vi "main.vi"() -> ()   [LabVIEW 2020]
uses:
  D:/SuperPython-master/ScintillaNET.dll
  ScintillaNET.dll
  <vilib>/picture/picture.llb/imagedata.ctl
  C:/Program Files/National Instruments/LabVIEW 2020/vi.lib/ActorFramework/Actor/Actor.lvclass
  <vilib>/ActorFramework/Message Enqueuer/Message Enqueuer.lvclass/Message Enqueuer.ctl
  <vilib>/ActorFramework/Message Enqueuer/Enqueue.vi
  C:/Program Files/National Instruments/LabVIEW 2020/vi.lib/ActorFramework/Message/Message.lvclass
  <vilib>/ActorFramework/Stop Msg/Stop Msg.lvclass
  <vilib>/ActorFramework/Message Priority Queue/Priority Enqueue.vi
  <vilib>/Utility/cursorutil.llb/Set Cursor (Icon Pict).vi
  <vilib>/Utility/inputDevices.llb/keyboardAcquire.vi
  <vilib>/Utility/inputDevices.llb/closeKeyboard.vi
  D:/SuperPython-master/AutocompleteMenu-ScintillaNET.dll
  AutocompleteMenu-ScintillaNET.dll
  <vilib>/ActorFramework/Actor/Actor.lvclass
panel:
  in  "工具-帮助":bool
  in  "菜单-下载":bool
  in  "切换界面":bool
  in  "工具-执行":bool
  in  "工具-编译":bool
  in  "工具-导出py":bool
  in  "工具-另存为":bool
  in  "工具-保存":bool
  in  "工具-新建":bool
  in  "工具-打开":bool
  in  "交互信息":string[][](array[string])
  in  "关键字":string[][](array[string])
  in  "执行语句":string[][](array[string])
  in  "图片名称":string[][](array[string])
  in  "停止":bool
  in  "界面":enum32{"选项卡 1", "选项卡 2"}(tab)
  out "编译执行状态":refnum<k24>(container) caption="文本程序"
  out "保存状态":string
  out "文本显示":refnum<k24>(container) caption="文本程序"
  in  "图形程序":picture[][](array[picture])
  out "备注":string[][](array[string])
  in  "辅助线":picture
  in  "连接线":picture
  in  "编辑控件类型":bool
  out "编辑控件":bool
  in  "控件类型":cluster{"二维图片":picture, "类型名称":string}[](array[cluster])
  in  "控件列表":T2(array[cluster])
  in  "全部控件":T3(array[cluster])
  in  "状态":refnum<k24>(container)
  in  "文本编辑":refnum<k24>(container)
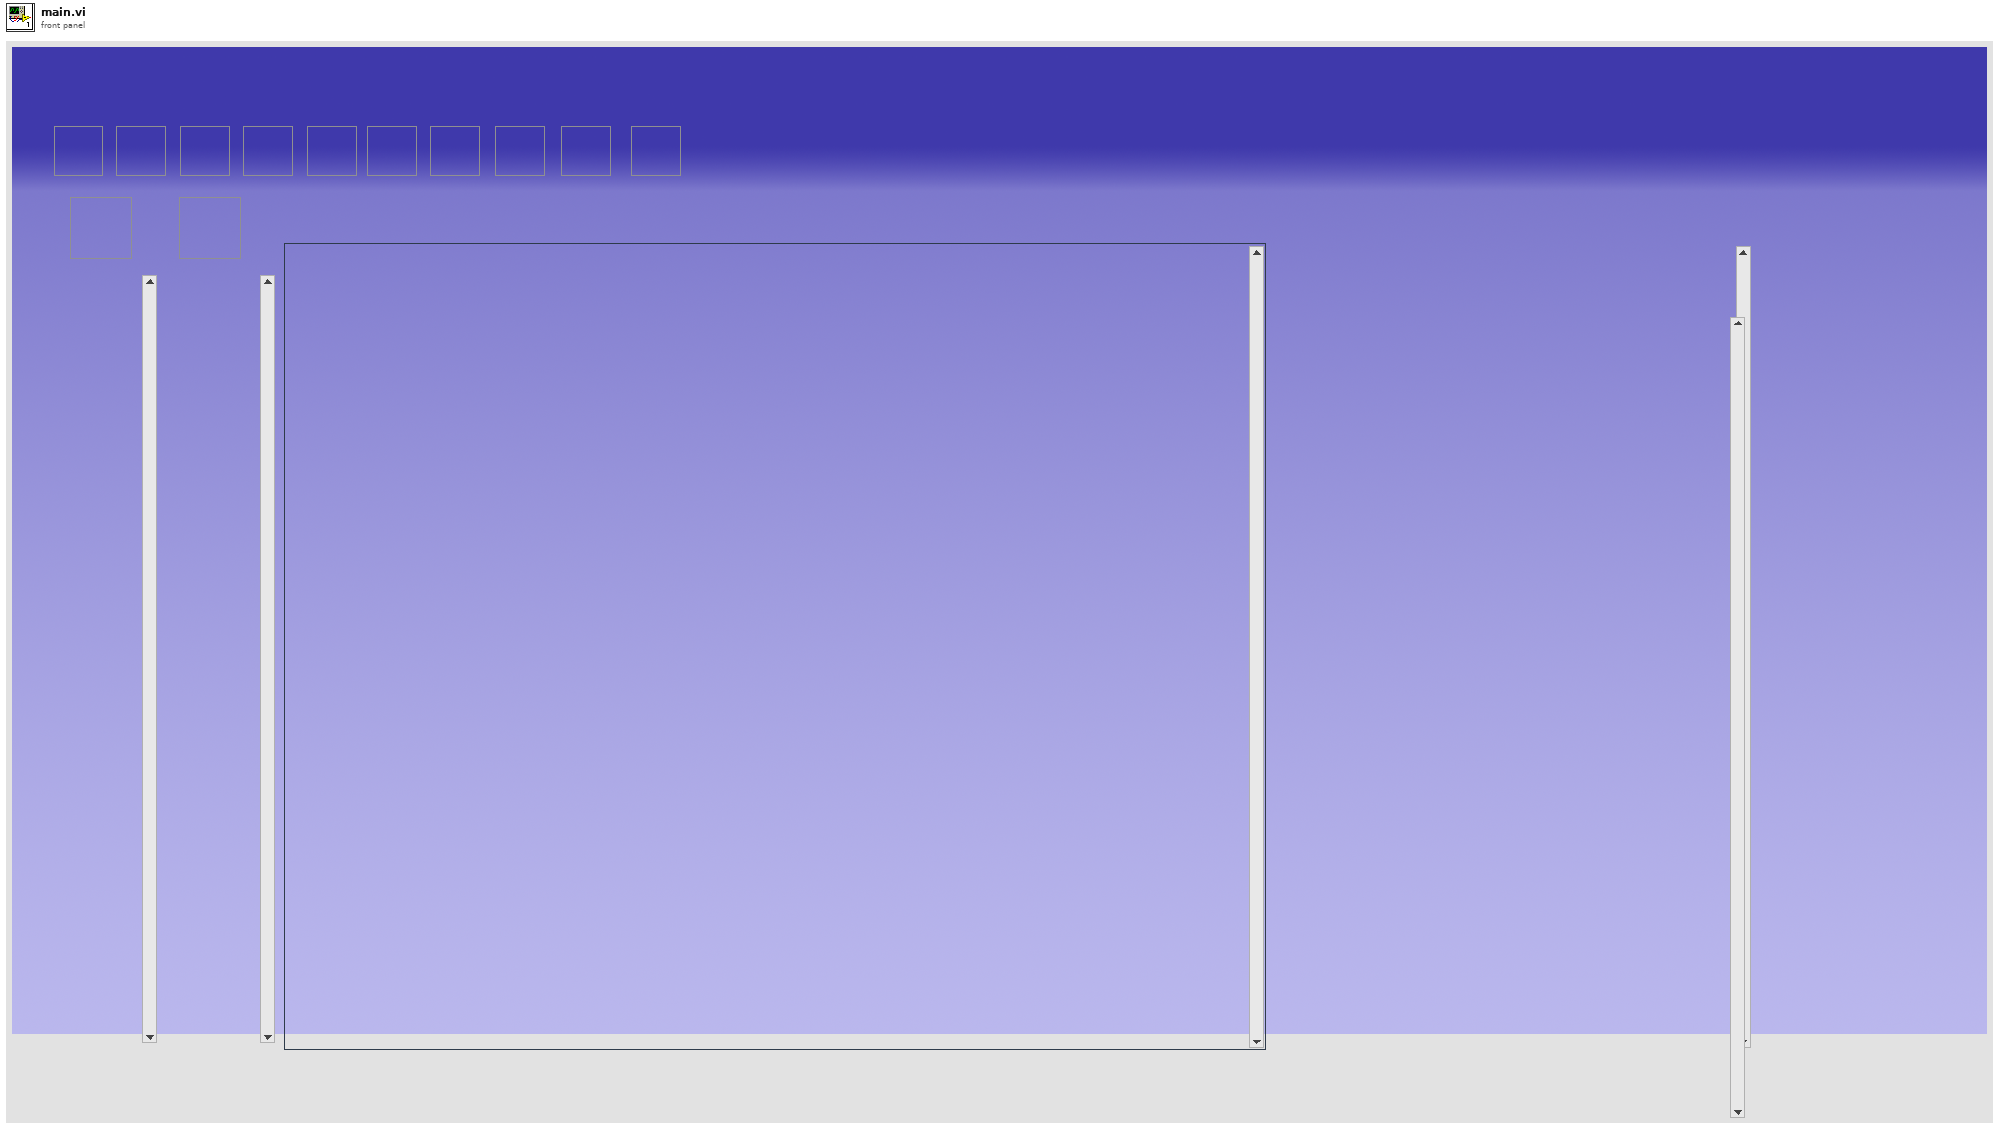
[diagram p1: front panel]
types:
  T1 = typedef "imagedata.ctl" = cluster{"image type":i32, "image depth":i32, "image":u8[], "mask":u8[], "colors":u32[], "Rectangle":cluster{"left":i16, "top":i16, "right":i16, "bottom":i16}}
  T2 = cluster{"图片":picture, "名称":string, "文本程序":string, "关键字":string, "image data":T1}[]
  T3 = cluster{"图片":picture, "名称":string, "文本程序":string, "关键字":string, "image data":T1}[][]
  T4 = cluster{"图形程序":refnum<vi>, "辅助线":refnum<vi>, "图片名称":refnum<vi>, "执行语句":refnum<vi>, "文本程序":refnum<vi>, "控件类型":refnum<vi>, "控件列表":refnum<vi>, "全部控件":refnum<vi>, "关键字":refnum<vi>, "连接线":refnum<vi>, "交互信息":refnum<vi>, "备注":refnum<vi>, "保存状态":refnum<vi>, "VI引用句柄":refnum<vi>, "编译执行状态":refnum<vi>, "TabCtl引用句柄":refnum<vi>, "AXContl":refnum<vi>, "AutoCompele":refnum<k24>, "状态":refnum<vi>}
  T5 = enum16{"0", "1", "2", "3", "4", "5", "6", "7", "8", "9", "A", "B", "C", "D", "E", "F", "G", "H", "I", "J", "K", "L", "M", "N", "O", "P", "Q", "R", "S", "T", "U", "V", "W", "X", "Y", "Z", "F1", "F2", "F3", "F4", "F5", "F6", "F7", "F8", "F9", "F10", "F11", "F12", "F13", "F14", "F15", "ADD", "BACK", "BACKSLASH", "CAPITAL", "COMMA", "DECIMAL", "DELETE", "DIVIDE", "DOWN", "END", "EQUALS", "ESCAPE", "GRAVE (`)", "HOME", "INSERT", "LBRACKET", "LCONTROL", "LEFT", "L ALT", "LSHIFT", "LWIN", "MINUS", "MULTIPLY", "NEXT", "NUMLOCK", "NUMPAD_0", "NUMPAD_1", "NUMPAD_2", "NUMPAD_3", "NUMPAD_4", "NUMPAD_5", "NUMPAD_6", "NUMPAD_7", "NUMPAD_8", "NUMPAD_9", "PAUSE", "PERIOD", "PRIOR (PG UP)", "RBRACKET", "RCONTROL", "RETURN", "RIGHT", "R ALT", "RSHIFT", "RWIN", "SCROLL", "SEMICOLON", "SLASH", "SPACE", "SUBTRACT", "TAB", "UP", "ENTER (num pad)", "' (quote)"}
  T6 = typedef "LVRectTypeDef.ctl" = cluster{"Left":i16, "Top":i16, "Right":i16, "Bottom":i16}
  T7 = typedef "LVPoint32TypeDef.ctl" = cluster{"Horizontal":i32, "Vertical":i32}
  T8 = typedef "LVPositionTypeDef.ctl" = cluster{"Left":i32, "Top":i32}
  T9 = typedef "eventvkey.ctl" = enum16{"ASCII", "Enter", "Return", "Shift", "Ctrl", "Alt", "Cmd", "Opt", "Caps", "NumLock", "Clear", "Break", "Up", "Down", "Left", "Right", "Insert", "Delete", "Home", "End", "PageUp", "PageDown", "Escape", "Help", "Pause", "ScrollLock", "F1", "F2", "F3", "F4", "F5", "F6", "F7", "F8", "F9", "F10", "F11", "F12", "F13", "F14", "F15", "F16", "F17", "F18", "F19", "F20", "F21", "F22", "F23", "F24", "Play", "VolumeUp", "VolumeDown", "Mute", "Two Byte Char"}
  T10 = enum16{"0", "1", "2", "3", "4", "5", "6", "7", "8", "9", "A", "B", "C", "D", "E", "F", "G", "H", "I", "J", "K", "L", "M", "N", "O", "P", "Q", "R", "S", "T", "U", "V", "W", "X", "Y", "Z", "F1", "F2", "F3", "F4", "F5", "F6", "F7", "F8", "F9", "F10", "F11", "F12", "F13", "F14", "F15", "ADD", "BACK", "BACKSLASH", "CAPITAL", "COMMA", "DECIMAL", "DELETE", "DIVIDE", "DOWN", "END", "EQUALS", "ESCAPE", "GRAVE (`)", "HOME", "INSERT", "LBRACKET", "LCONTROL", "LEFT", "L ALT", "LSHIFT", "LWIN", "MINUS", "MULTIPLY", "NEXT", "NUMLOCK", "NUMPAD_0", "NUMPAD_1", "NUMPAD_2", "NUMPAD_3", "NUMPAD_4", "NUMPAD_5", "NUMPAD_6", "NUMPAD_7", "NUMPAD_8", "NUMPAD_9", "PAUSE", "PERIOD", "PRIOR (PG UP)", "RBRACKET", "RCONTROL", "RETURN", "RIGHT", "R ALT", "RSHIFT", "RWIN", "SCROLL", "SEMICOLON", "SLASH", "SPACE", "SUBTRACT", "TAB", "UP", "ENTER (num pad)", "' (quote)"}[]
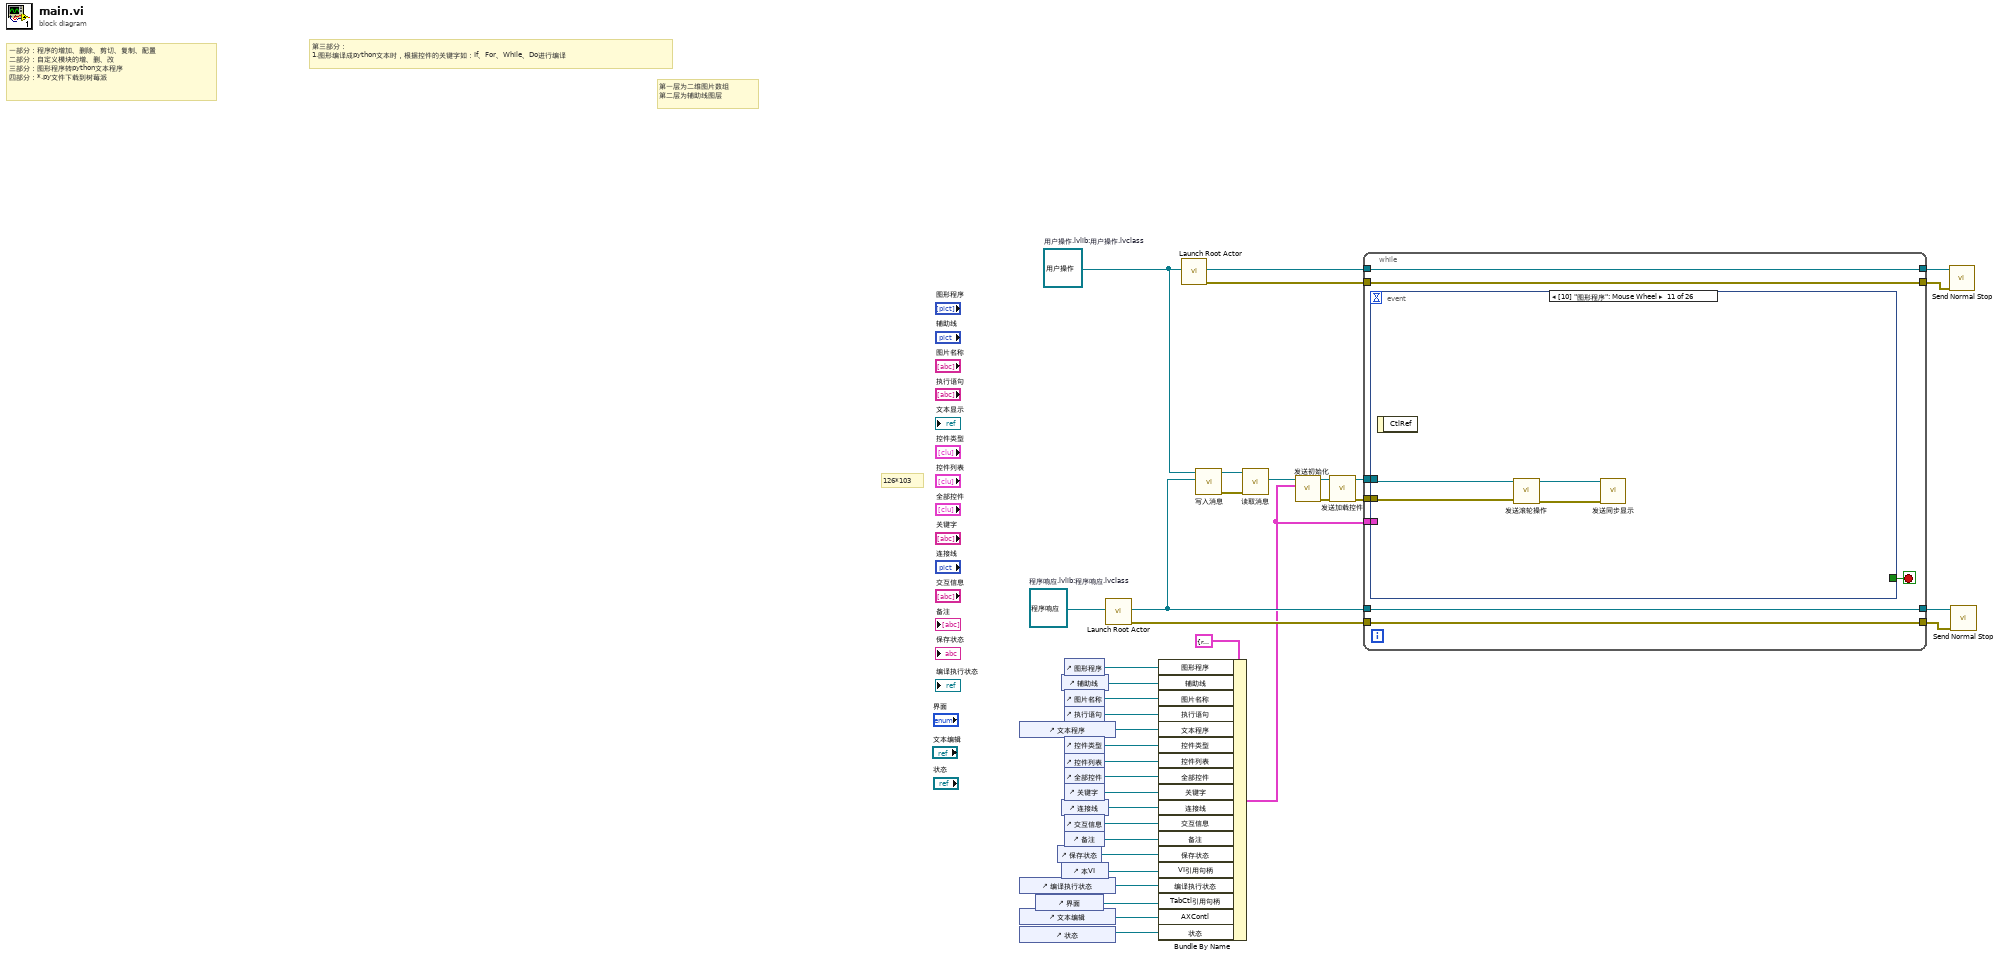
[diagram p0: block diagram]
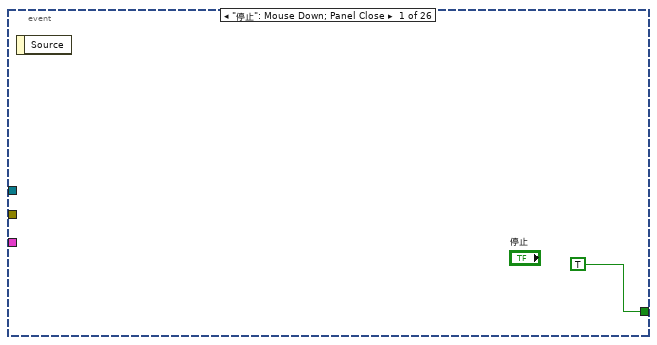
[diagram p2: hidden frame]
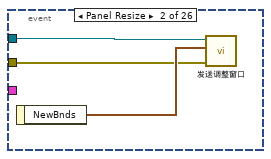
[diagram p3: hidden frame]
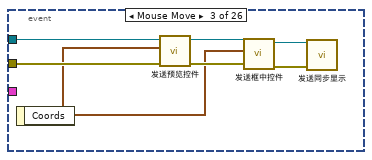
[diagram p4: hidden frame]
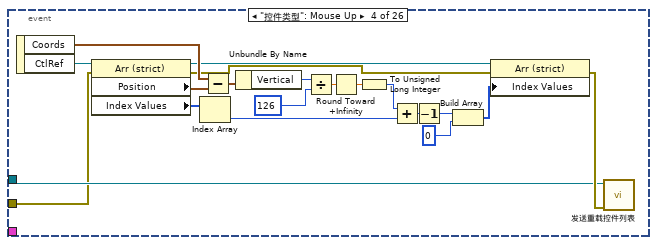
[diagram p5: hidden frame]
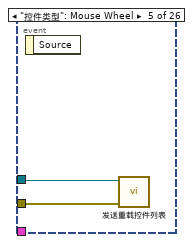
[diagram p6: hidden frame]
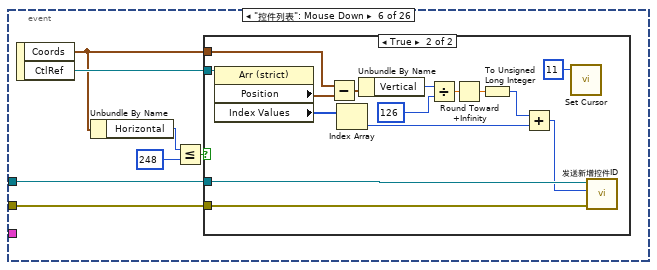
[diagram p7: hidden frame]
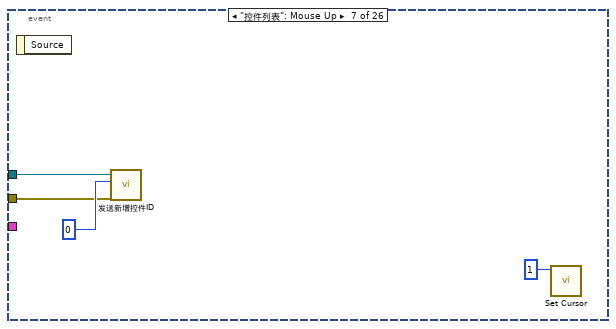
[diagram p9: hidden frame]
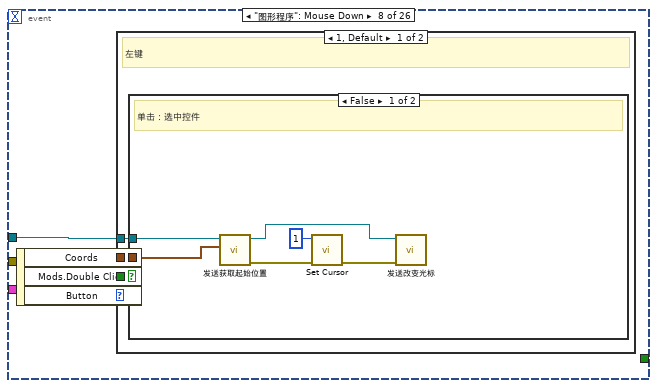
[diagram p10: hidden frame]
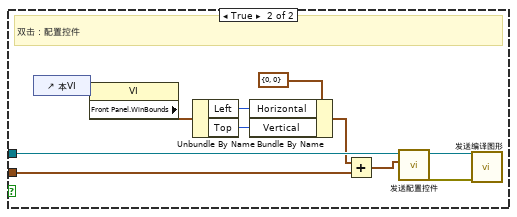
[diagram p11: hidden frame]
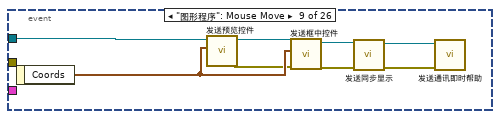
[diagram p13: hidden frame]
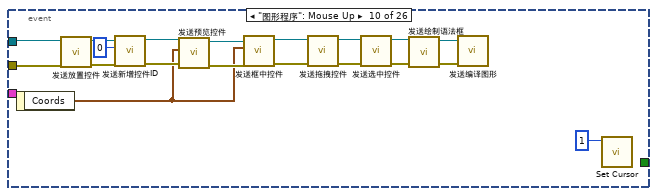
[diagram p14: hidden frame]
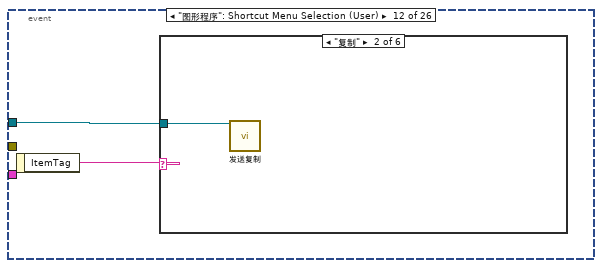
[diagram p15: hidden frame]
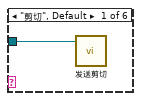
[diagram p16: hidden frame]
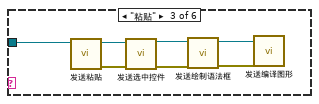
[diagram p17: hidden frame]
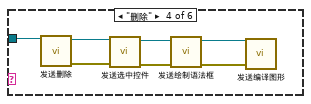
[diagram p18: hidden frame]
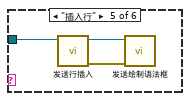
[diagram p19: hidden frame]
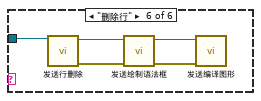
[diagram p20: hidden frame]
diagram:
  w34 = refnum<class "用户操作.lvclass"> refnum  # 用户操作.lvlib:用户操作.lvclass
  w37 = refnum<class "程序响应.lvclass"> refnum  # 程序响应.lvlib:程序响应.lvclass
  # "126*103"
  # "第三部分：\n1.图形编译成python文本时，根据控件的关键字如：If、For、While、Do进行编译"
  # "一部分：程序的增加、删除、剪切、复制、配置\n二部分：自定义模块的增、删、改\n三部分：图形程序转python文本程序\n四部分：*.py文件下载到树莓派"
  # "第一层为二维图片数组\n第二层为辅助线图层"
  n1 = control-ref of="文本程序"() -> (w21:refnum<vi>)
  n2 = control-ref of="编译执行状态"() -> (w13:refnum<vi>)
  n3 = control-ref of="文本编辑"() -> (w10:refnum<vi>)
  n4 = control-ref of="状态"() -> (w5:refnum<vi>)
  n5 = control-ref of="界面"() -> (w11:refnum<vi>)
  n6 = control-ref of="保存状态"() -> (w15:refnum<vi>)
  n7 = control-ref of="辅助线"() -> (w24:refnum<vi>)
  n8 = control-ref of="连接线"() -> (w19:refnum<vi>)
  n9 = control-ref of="本VI"() -> (w14:refnum<vi>)
  n10 = control-ref of="图形程序"() -> (w25:refnum<vi>)
  n11 = control-ref of="图片名称"() -> (w23:refnum<vi>)
  n12 = control-ref of="执行语句"() -> (w22:refnum<vi>)
  n13 = control-ref of="控件类型"() -> (w18:refnum<vi>)
  n14 = control-ref of="控件列表"() -> (w3:refnum<vi>)
  n15 = control-ref of="全部控件"() -> (w2:refnum<vi>)
  n16 = control-ref of="关键字"() -> (w20:refnum<vi>)
  n17 = control-ref of="交互信息"() -> (w17:refnum<vi>)
  n18 = control-ref of="备注"() -> (w16:refnum<vi>)
  n19 = call <vilib>:"Launch Root Actor.vi"("Actor"=w37) -> ("error out"=w29:errorcluster, "Actor's Enqueuer"=w33:refnum<class "Message Enqueuer.lvclass">)  [unwired: 9 in]
  n20 = Bundle By Name(cluster=T4 {"图形程序"=refnum, "辅助线"=refnum, "图片名称"=refnum, "执行语句"=refnum, "文本程序"=refnum, "控件类型"=refnum, "控件列表"=refnum, "全部控件"=refnum, "关键字"=refnum, "连接线"=refnum, "交互信息"=refnum, "备注"=refnum, "保存状态"=refnum, "VI引用句柄"=refnum, "编译执行状态"=refnum, "TabCtl引用句柄"=refnum, "AXContl"=refnum, "AutoCompele"=refnum, "状态"=refnum} ("数据"), "图形程序"=w25, "辅助线"=w24, "图片名称"=w23, "执行语句"=w22, "文本程序"=w21, "控件类型"=w18, "控件列表"=w3, "全部控件"=w2, "关键字"=w20, "连接线"=w19, "交互信息"=w17, "备注"=w16, "保存状态"=w15, "VI引用句柄"=w14, "编译执行状态"=w13, "TabCtl引用句柄"=w11, "AXContl"=w10, "状态"=w5) -> (w1:T4)
  n21 = call <vilib>:"Launch Root Actor.vi"("Actor"=w34) -> ("error out"=w27:errorcluster, "Actor's Enqueuer"=w32:refnum<class "Message Enqueuer.lvclass">)  [unwired: 9 in]
  n22 = call-dynamic "写入消息.vi"("操作者框架:消息待入队列"=w33, "用户操作输入"=w34) -> ("error out"=w35:errorcluster, "用户操作输出"=w36:refnum<class "用户操作.lvclass">)  [unwired: 8 in]
  n23 = call-dynamic "读取消息.vi"("error in (no error)"=w35, "用户操作输入"=w36) -> ("操作者框架:消息待入队列"=w12:refnum<class "Message Enqueuer.lvclass">)  [unwired: 7 in, 2 out]
  n24 = call "发送初始化.vi"("数据"=w1, "Message Enqueuer"=w12) -> ("error out"=w7:errorcluster, "Message Enqueuer out"=w9:refnum<class "Message Enqueuer.lvclass">)  [unwired: 8 in]
  n25 = call "发送加载控件.vi"("error in (no error)"=w7, "Message Enqueuer"=w9) -> ("error out"=w6:errorcluster, "Message Enqueuer out"=w8:refnum<class "Message Enqueuer.lvclass">)  [unwired: 8 in]
  n26 = while {
    tunnel: w33 -> [w43]
    tunnel: w8 -> [w45]
    tunnel: w32 -> [w44]
    tunnel: [w44] -> w31
    tunnel: [w43] -> w30
    tunnel: w29 -> [w42]
    tunnel: [w42] -> w28
    tunnel: w27 -> [w41]
    tunnel: [w41] -> w26
    tunnel: w1 -> [w39]
    tunnel: w6 -> [w38]
    stop <- w40 stop-if-true
    n27 = event shown="[10] \"图形程序\": Mouse Wheel" {
      selector: _ -> [_ _ _ _ _ _ _ _ _ _ _ _ _ _ _ _ _ _ _ _ _ _ _ _ _ _]
      dyn-events: _ -> [_ _ _ _ _ _ _ _ _ _ _ _ _ _ _ _ _ _ _ _ _ _ _ _ _ _]
      timeout: _ -> [_ _ _ _ _ _ _ _ _ _ _ _ _ _ _ _ _ _ _ _ _ _ _ _ _ _]
      tunnel: w45 -> [_ w49 w54 w59 w78 w85 w104 w108 w136 w152 w158 w160 w186 w212 w215 w217 w222 w223 w224 w226 w227 w228 w230 w231 w234 w248]
      tunnel: [TRUE _ _ _ _ _ _ _ _ _ _ _ _ _ _ _ _ _ _ _ _ _ _ _ _ _] -> w40
      tunnel: w39 -> [_ _ _ _ _ _ _ _ _ _ _ _ _ _ _ w216 _ _ _ _ _ _ _ _ _ _]
      tunnel: w38 -> [_ w47 w53 w58 w77 w83 w101 _ _ w137 w156 _ _ _ _ _ _ _ _ _ _ _ _ _ _ w247]
      event "停止": Mouse Down; Panel Close {
        n28 = event-data() -> ()  [unwired: 1 in, 1 out]
      }
      event Panel Resize {
        n29 = event-data() -> ("NewBnds"=w48:T6)  [unwired: 1 in]
        n30 = call "发送调整窗口.vi"("error in (no error)"=w47, "前面板范围"=w48, "Message Enqueuer"=w49) -> ()  [unwired: 7 in, 2 out]
      }
      event Mouse Move {
        n31 = event-data() -> ("Coords"=w50:T7)  [unwired: 1 in]
        n32 = call "发送预览控件.vi"("error in (no error)"=w53, "鼠标位置"=w50, "Message Enqueuer"=w54) -> ("error out"=w52:errorcluster, "Message Enqueuer out"=w56:refnum<class "Message Enqueuer.lvclass">)  [unwired: 7 in]
        n33 = call "发送框中控件.vi"("error in (no error)"=w52, "结束坐标"=w50, "Message Enqueuer"=w56) -> ("error out"=w51:errorcluster, "Message Enqueuer out"=w55:refnum<class "Message Enqueuer.lvclass">)  [unwired: 7 in]
        n34 = call "发送同步显示.vi"("error in (no error)"=w51, "Message Enqueuer"=w55) -> ()  [unwired: 8 in, 2 out]
      }
      event "控件类型": Mouse Up {
        n35 = event-data() -> ("Coords"=w67:T7, "CtlRef"=w66:refnum<vi>)  [unwired: 1 in]
        n36 = property class="Arr (strict)"(reference=w66, error in=w58) -> (reference out=w65:refnum<vi>, error out=w57:errorcluster, "Position"=w76:T8, "Index Values"=w71:u32[])
        n37 = Index Array(array=w71) -> (element=w70:u32)  [unwired: 1 in]
        n38 = Subtract(x=w67, y=w76) -> (x-y=w75:T7)
        n39 = Unbundle By Name(w75) -> ("Vertical"=w74:i32)
        n40 = Divide(x=w74, y=126) -> (x/y=w72:dbl)
        n41 = Round Toward +Infinity(x=w72) -> (ceil(x): smallest int >= x=w69:dbl)
        n42 = To Unsigned Long Integer(number=w69) -> (unsigned 32bit integer=w68:u32)
        n43 = Add(x=w68, y=w70) -> (x+y=w64:u32)
        n44 = Decrement(x=w64) -> (x-1=w61:u32)
        n45 = Build Array(w61, u32 0 ("元素")) -> (w62:u32[])
        n46 = property class="Arr (strict)"(reference=w65, error in=w57, "Index Values"=w62) -> (error out=w60:errorcluster)  [unwired: 1 out]
        n47 = call "发送重载控件列表.vi"("error in (no error)"=w60, "Message Enqueuer"=w59) -> ()  [unwired: 8 in, 2 out]
      }
      event "控件类型": Mouse Wheel {
        n48 = event-data() -> ()  [unwired: 1 in, 1 out]
        n49 = call "发送重载控件列表.vi"("error in (no error)"=w77, "Message Enqueuer"=w78) -> ()  [unwired: 8 in, 2 out]
      }
      event "控件列表": Mouse Down {
        n50 = event-data() -> ("Coords"=w82:T7, "CtlRef"=w84:refnum<vi>)  [unwired: 1 in]
        n51 = Unbundle By Name(w82) -> ("Horizontal"=w81:i32)
        n52 = Less Or Equal?(x=w81, y=248) -> (x <= y?=w80:bool)
        n53 = case shown="True" w80 {
          tunnel: w85 -> [_ w91]
          tunnel: w84 -> [_ w90]
          tunnel: w82 -> [_ w88]
          tunnel: w83 -> [_ w87]
          frame False {
          }
          frame True {
            n54 = property class="Arr (strict)"(reference=w90) -> ("Position"=w100:T8, "Index Values"=w95:u32[])  [unwired: 1 in, 2 out]
            n55 = Subtract(x=w88, y=w100) -> (x-y=w99:T7)
            n56 = Index Array(array=w95) -> (element=w94:u32)  [unwired: 1 in]
            n57 = Unbundle By Name(w99) -> ("Vertical"=w98:i32)
            n58 = Divide(x=w98, y=126) -> (x/y=w96:dbl)
            n59 = Round Toward +Infinity(x=w96) -> (ceil(x): smallest int >= x=w93:dbl)
            n60 = To Unsigned Long Integer(number=w93) -> (unsigned 32bit integer=w92:u32)
            n61 = Add(x=w92, y=w94) -> (x+y=w89:u32)
            n62 = call-poly <vilib>:"Set Cursor.vi"("icon"=u16 11) -> ()  [unwired: 9 in, 2 out]
            n63 = call "发送新增控件ID.vi"("error in (no error)"=w87, "控件ID"=w89, "Message Enqueuer"=w91) -> ()  [unwired: 7 in, 2 out]
          }
        }
      }
      event "控件列表": Mouse Up {
        n64 = event-data() -> ()  [unwired: 1 in, 1 out]
        n65 = call "发送新增控件ID.vi"("error in (no error)"=w101, "控件ID"=u32 0, "Message Enqueuer"=w104) -> ()  [unwired: 7 in, 2 out]
        n66 = call-poly <vilib>:"Set Cursor.vi"("icon"=u16 1) -> ()  [unwired: 9 in, 2 out]
      }
      event "图形程序": Mouse Down {
        n67 = event-data() -> ("Coords"=w107:T7, "Mods.Double Click"=w105:bool, "Button"=w106:u16)  [unwired: 1 in]
        n68 = case shown="1, Default" w106 {
          tunnel: w108 -> [w111 _]
          tunnel: w107 -> [w110 _]
          tunnel: w105 -> [w109 _]
          frame 1, Default {
            # "左键"
            n69 = case shown="False" w109 {
              tunnel: w111 -> [w117 w128]
              tunnel: w110 -> [w116 w126]
              frame False {
                # "单击：选中控件"
                n70 = call "发送获取起始位置.vi"("起始坐标"=w116, "Message Enqueuer"=w117) -> ("error out"=w114:errorcluster, "Message Enqueuer out"=w112:refnum<class "Message Enqueuer.lvclass">)  [unwired: 8 in]
                n71 = call-poly <vilib>:"Set Cursor.vi"("error in (no error)"=w114, "icon"=u16 1) -> ("error out"=w113:errorcluster)  [unwired: 8 in, 1 out]
                n72 = call "发送改变光标.vi"("error in (no error)"=w113, "Message Enqueuer"=w112) -> ()  [unwired: 8 in, 2 out]
              }
              frame True {
                # "双击：配置控件"
                n73 = control-ref of="本VI"() -> (w127:refnum<vi>)
                n74 = property class="VI"(reference=w127) -> ("Front Panel.WinBounds"=w124:T6)  [unwired: 1 in, 2 out]
                n75 = Unbundle By Name(w124) -> ("Left"=w123:i16, "Top"=w122:i16)
                n76 = Bundle By Name(cluster=cluster{"Horizontal":i32, "Vertical":i32} {"Horizontal"=0, "Vertical"=0} ("x"), "Horizontal"=w123, "Vertical"=w122) -> (w120:cluster{"Horizontal":i32, "Vertical":i32})
                n77 = Add(x=w120, y=w126) -> (x+y=w125:T7)
                n78 = call "发送配置控件.vi"("鼠标位置"=w125, "Message Enqueuer"=w128) -> ("error out"=w118:errorcluster, "Message Enqueuer out"=w119:refnum<class "Message Enqueuer.lvclass">)  [unwired: 8 in]
                n79 = call "发送编译图形.vi"("error in (no error)"=w118, "Message Enqueuer"=w119) -> ()  [unwired: 8 in, 2 out]
              }
            }
          }
          frame 2 {
            # "右键自定义菜单"
          }
        }
      }
      event "图形程序": Mouse Move {
        n80 = event-data() -> ("Coords"=w134:T7)  [unwired: 1 in]
        n81 = call "发送预览控件.vi"("鼠标位置"=w134, "Message Enqueuer"=w136) -> ("error out"=w133:errorcluster, "Message Enqueuer out"=w135:refnum<class "Message Enqueuer.lvclass">)  [unwired: 8 in]
        n82 = call "发送框中控件.vi"("error in (no error)"=w133, "结束坐标"=w134, "Message Enqueuer"=w135) -> ("error out"=w131:errorcluster, "Message Enqueuer out"=w132:refnum<class "Message Enqueuer.lvclass">)  [unwired: 7 in]
        n83 = call "发送同步显示.vi"("error in (no error)"=w131, "Message Enqueuer"=w132) -> ("error out"=w129:errorcluster, "Message Enqueuer out"=w130:refnum<class "Message Enqueuer.lvclass">)  [unwired: 8 in]
        n84 = call "发送通讯即时帮助.vi"("error in (no error)"=w129, "Message Enqueuer"=w130) -> ()  [unwired: 8 in, 2 out]
      }
      event "图形程序": Mouse Up {
        n85 = event-data() -> ("Coords"=w147:T7)  [unwired: 1 in]
        n86 = call "发送放置控件.vi"("error in (no error)"=w137, "Message Enqueuer"=w152) -> ("error out"=w153:errorcluster, "Message Enqueuer out"=w154:refnum<class "Message Enqueuer.lvclass">)  [unwired: 8 in]
        n87 = call "发送新增控件ID.vi"("error in (no error)"=w153, "控件ID"=u32 0, "Message Enqueuer"=w154) -> ("error out"=w150:errorcluster, "Message Enqueuer out"=w151:refnum<class "Message Enqueuer.lvclass">)  [unwired: 7 in]
        n88 = call "发送预览控件.vi"("error in (no error)"=w150, "鼠标位置"=w147, "Message Enqueuer"=w151) -> ("error out"=w148:errorcluster, "Message Enqueuer out"=w149:refnum<class "Message Enqueuer.lvclass">)  [unwired: 7 in]
        n89 = call "发送框中控件.vi"("error in (no error)"=w148, "结束坐标"=w147, "Message Enqueuer"=w149) -> ("error out"=w140:errorcluster, "Message Enqueuer out"=w141:refnum<class "Message Enqueuer.lvclass">)  [unwired: 7 in]
        n90 = call "发送拖拽控件.vi"("error in (no error)"=w140, "Message Enqueuer"=w141) -> ("error out"=w138:errorcluster, "Message Enqueuer out"=w139:refnum<class "Message Enqueuer.lvclass">)  [unwired: 8 in]
        n91 = call "发送选中控件.vi"("error in (no error)"=w138, "Message Enqueuer"=w139) -> ("error out"=w142:errorcluster, "Message Enqueuer out"=w143:refnum<class "Message Enqueuer.lvclass">)  [unwired: 8 in]
        n92 = call "发送绘制语法框.vi"("error in (no error)"=w142, "Message Enqueuer"=w143) -> ("error out"=w144:errorcluster, "Message Enqueuer out"=w145:refnum<class "Message Enqueuer.lvclass">)  [unwired: 8 in]
        n93 = call "发送编译图形.vi"("error in (no error)"=w144, "Message Enqueuer"=w145) -> ()  [unwired: 8 in, 2 out]
        n94 = call-poly <vilib>:"Set Cursor.vi"("icon"=u16 1) -> ()  [unwired: 9 in, 2 out]
      }
      event "图形程序": Mouse Wheel {
        n95 = event-data() -> ()  [unwired: 1 in, 1 out]
        n96 = call "发送滚轮操作.vi"("error in (no error)"=w156, "Message Enqueuer"=w158) -> ("error out"=w157:errorcluster, "Message Enqueuer out"=w159:refnum<class "Message Enqueuer.lvclass">)  [unwired: 8 in]
        n97 = call "发送同步显示.vi"("error in (no error)"=w157, "Message Enqueuer"=w159) -> ()  [unwired: 8 in, 2 out]
      }
      event "图形程序": Shortcut Menu Selection (User) {
        n98 = event-data() -> ("ItemTag"=w161:string)  [unwired: 1 in]
        n99 = case shown="\"复制\"" w161 {
          tunnel: w160 -> [w162 w163 w170 w177 w180 w185]
          frame "剪切", Default {
            n100 = call "发送剪切.vi"("Message Enqueuer"=w162) -> ()  [unwired: 9 in, 2 out]
          }
          frame "复制" {
            n101 = call "发送复制.vi"("Message Enqueuer"=w163) -> ()  [unwired: 9 in, 2 out]
          }
          frame "粘贴" {
            n102 = call "发送粘贴.vi"("Message Enqueuer"=w170) -> ("error out"=w166:errorcluster, "Message Enqueuer out"=w169:refnum<class "Message Enqueuer.lvclass">)  [unwired: 9 in]
            n103 = call "发送选中控件.vi"("error in (no error)"=w166, "Message Enqueuer"=w169) -> ("error out"=w165:errorcluster, "Message Enqueuer out"=w168:refnum<class "Message Enqueuer.lvclass">)  [unwired: 8 in]
            n104 = call "发送绘制语法框.vi"("error in (no error)"=w165, "Message Enqueuer"=w168) -> ("error out"=w164:errorcluster, "Message Enqueuer out"=w167:refnum<class "Message Enqueuer.lvclass">)  [unwired: 8 in]
            n105 = call "发送编译图形.vi"("error in (no error)"=w164, "Message Enqueuer"=w167) -> ()  [unwired: 8 in, 2 out]
          }
          frame "删除" {
            n106 = call "发送删除.vi"("Message Enqueuer"=w177) -> ("error out"=w173:errorcluster, "Message Enqueuer out"=w176:refnum<class "Message Enqueuer.lvclass">)  [unwired: 9 in]
            n107 = call "发送选中控件.vi"("error in (no error)"=w173, "Message Enqueuer"=w176) -> ("error out"=w172:errorcluster, "Message Enqueuer out"=w175:refnum<class "Message Enqueuer.lvclass">)  [unwired: 8 in]
            n108 = call "发送绘制语法框.vi"("error in (no error)"=w172, "Message Enqueuer"=w175) -> ("error out"=w171:errorcluster, "Message Enqueuer out"=w174:refnum<class "Message Enqueuer.lvclass">)  [unwired: 8 in]
            n109 = call "发送编译图形.vi"("error in (no error)"=w171, "Message Enqueuer"=w174) -> ()  [unwired: 8 in, 2 out]
          }
          frame "插入行" {
            n110 = call "发送行插入.vi"("Message Enqueuer"=w180) -> ("error out"=w178:errorcluster, "Message Enqueuer out"=w179:refnum<class "Message Enqueuer.lvclass">)  [unwired: 9 in]
            n111 = call "发送绘制语法框.vi"("error in (no error)"=w178, "Message Enqueuer"=w179) -> ()  [unwired: 8 in, 2 out]
          }
          frame "删除行" {
            n112 = call "发送行删除.vi"("Message Enqueuer"=w185) -> ("error out"=w182:errorcluster, "Message Enqueuer out"=w184:refnum<class "Message Enqueuer.lvclass">)  [unwired: 9 in]
            n113 = call "发送绘制语法框.vi"("error in (no error)"=w182, "Message Enqueuer"=w184) -> ("error out"=w181:errorcluster, "Message Enqueuer out"=w183:refnum<class "Message Enqueuer.lvclass">)  [unwired: 8 in]
            n114 = call "发送编译图形.vi"("error in (no error)"=w181, "Message Enqueuer"=w183) -> ()  [unwired: 8 in, 2 out]
          }
        }
      }
      event Key Down {
        n115 = event-data() -> ("PlatMods.Ctrl"=w189:bool, "Char"=w188:i16, "VKey"=w187:T9)  [unwired: 1 in]
        n116 = case shown="True" w189 {
          tunnel: w188 -> [_ w197]
          tunnel: w187 -> [w191 _]
          tunnel: w186 -> [w190 w196]
          frame False {
            n117 = case shown="\"Delete\"" w191 {
              tunnel: w190 -> [_ w194]
              frame "ASCII", Default {
              }
              frame "Delete" {
                # "删除"
                n118 = call "发送删除.vi"("Message Enqueuer"=w194) -> ("Message Enqueuer out"=w195:refnum<class "Message Enqueuer.lvclass">)  [unwired: 9 in, 1 out]
                n119 = call "发送选中控件.vi"("Message Enqueuer"=w195) -> ("Message Enqueuer out"=w193:refnum<class "Message Enqueuer.lvclass">)  [unwired: 9 in, 1 out]
                n120 = call "发送绘制语法框.vi"("Message Enqueuer"=w193) -> ("Message Enqueuer out"=w192:refnum<class "Message Enqueuer.lvclass">)  [unwired: 9 in, 1 out]
                n121 = call "发送编译图形.vi"("Message Enqueuer"=w192) -> ()  [unwired: 9 in, 2 out]
              }
            }
          }
          frame True {
            n122 = case shown="118" w197 {
              tunnel: w196 -> [_ w198 w202 w203 w204 w207 w209]
              frame 0, Default {
              }
              frame 99 {
                # "复制"
                n123 = call "发送复制.vi"("Message Enqueuer"=w198) -> ()  [unwired: 9 in, 2 out]
              }
              frame 118 {
                # "粘贴"
                n124 = call "发送粘贴.vi"("Message Enqueuer"=w202) -> ("Message Enqueuer out"=w201:refnum<class "Message Enqueuer.lvclass">)  [unwired: 9 in, 1 out]
                n125 = call "发送选中控件.vi"("Message Enqueuer"=w201) -> ("Message Enqueuer out"=w200:refnum<class "Message Enqueuer.lvclass">)  [unwired: 9 in, 1 out]
                n126 = call "发送绘制语法框.vi"("Message Enqueuer"=w200) -> ("Message Enqueuer out"=w199:refnum<class "Message Enqueuer.lvclass">)  [unwired: 9 in, 1 out]
                n127 = call "发送编译图形.vi"("Message Enqueuer"=w199) -> ()  [unwired: 9 in, 2 out]
              }
              frame 120 {
                # "剪切"
                n128 = call "发送剪切.vi"("Message Enqueuer"=w203) -> ()  [unwired: 9 in, 2 out]
              }
              frame 97 {
                # "CTRL+A插入行"
                n129 = call "发送行插入.vi"("Message Enqueuer"=w204) -> ("Message Enqueuer out"=w205:refnum<class "Message Enqueuer.lvclass">)  [unwired: 9 in, 1 out]
                n130 = call "发送绘制语法框.vi"("Message Enqueuer"=w205) -> ()  [unwired: 9 in, 2 out]
              }
              frame 100 {
                # "CTRL+D删除行"
                n131 = call "发送行删除.vi"("Message Enqueuer"=w207) -> ("Message Enqueuer out"=w208:refnum<class "Message Enqueuer.lvclass">)  [unwired: 9 in, 1 out]
                n132 = call "发送绘制语法框.vi"("Message Enqueuer"=w208) -> ("Message Enqueuer out"=w206:refnum<class "Message Enqueuer.lvclass">)  [unwired: 9 in, 1 out]
                n133 = call "发送编译图形.vi"("Message Enqueuer"=w206) -> ()  [unwired: 9 in, 2 out]
              }
              frame 115 {
                # "保存文件"
                n134 = call "发送菜单-保存.vi"("Message Enqueuer"=w209) -> ()  [unwired: 9 in, 2 out]
              }
            }
          }
        }
      }
      event "编辑控件类型": Mouse Up {
        n135 = event-data() -> ()  [unwired: 1 in, 1 out]
        n136 = call "发送编辑控件类型.vi"("Message Enqueuer"=w212) -> ("error out"=w210:errorcluster, "Message Enqueuer out"=w211:refnum<class "Message Enqueuer.lvclass">)  [unwired: 9 in]
        n137 = call "发送加载控件.vi"("error in (no error)"=w210, "Message Enqueuer"=w211) -> ()  [unwired: 8 in, 2 out]
      }
      event "编辑控件": Mouse Up {
        n138 = event-data() -> ()  [unwired: 1 in, 1 out]
        n139 = call "发送编辑控件.vi"("Message Enqueuer"=w215) -> ("error out"=w213:errorcluster, "Message Enqueuer out"=w214:refnum<class "Message Enqueuer.lvclass">)  [unwired: 9 in]
        n140 = call "发送加载控件.vi"("error in (no error)"=w213, "Message Enqueuer"=w214) -> ()  [unwired: 8 in, 2 out]
      }
      event "工具-新建": Mouse Up {
        n141 = event-data() -> ()  [unwired: 1 in, 1 out]
        n142 = call "发送初始化.vi"("数据"=w216, "Message Enqueuer"=w217) -> ()  [unwired: 8 in, 2 out]
      }
      event "工具-打开": Mouse Up {
        n143 = event-data() -> ()  [unwired: 1 in, 1 out]
        n144 = call "发送菜单-打开.vi"("Message Enqueuer"=w222) -> ("error out"=w218:errorcluster, "Message Enqueuer out"=w221:refnum<class "Message Enqueuer.lvclass">)  [unwired: 9 in]
        n145 = call "发送绘制语法框.vi"("error in (no error)"=w218, "Message Enqueuer"=w221) -> ("error out"=w219:errorcluster, "Message Enqueuer out"=w220:refnum<class "Message Enqueuer.lvclass">)  [unwired: 8 in]
        n146 = call "发送编译图形.vi"("error in (no error)"=w219, "Message Enqueuer"=w220) -> ()  [unwired: 8 in, 2 out]
      }
      event "工具-保存": Mouse Up {
        n147 = event-data() -> ()  [unwired: 1 in, 1 out]
        n148 = call "发送菜单-保存.vi"("Message Enqueuer"=w223) -> ()  [unwired: 9 in, 2 out]
      }
      event "工具-另存为": Mouse Up {
        n149 = event-data() -> ()  [unwired: 1 in, 1 out]
        n150 = call "发送菜单-另存为.vi"("Message Enqueuer"=w224) -> ()  [unwired: 9 in, 2 out]
      }
      event "工具-导出py": Mouse Up {
        n151 = event-data() -> ()  [unwired: 1 in, 1 out]
        n152 = call "发送编译图形.vi"("Message Enqueuer"=w226) -> ("Message Enqueuer out"=w225:refnum<class "Message Enqueuer.lvclass">)  [unwired: 9 in, 1 out]
        n153 = call "发送菜单-导出py.vi"("Message Enqueuer"=w225) -> ()  [unwired: 9 in, 2 out]
      }
      event "工具-编译": Mouse Up {
        n154 = event-data() -> ()  [unwired: 1 in, 1 out]
        n155 = call "发送菜单-编译.vi"("Message Enqueuer"=w227) -> ()  [unwired: 9 in, 2 out]
      }
      event "工具-执行": Mouse Up {
        n156 = event-data() -> ()  [unwired: 1 in, 1 out]
        n157 = call "发送菜单-执行.vi"("Message Enqueuer"=w228) -> ()  [unwired: 9 in, 2 out]
      }
      event "菜单-下载": Mouse Up {
        n158 = event-data() -> ()  [unwired: 1 in, 1 out]
        n159 = call "发送编译图形.vi"("Message Enqueuer"=w230) -> ("Message Enqueuer out"=w229:refnum<class "Message Enqueuer.lvclass">)  [unwired: 9 in, 1 out]
        n160 = call "发送菜单-下载.vi"("Message Enqueuer"=w229) -> ()  [unwired: 9 in, 2 out]
      }
      event "工具-帮助": Mouse Up {
        n161 = event-data() -> ()  [unwired: 1 in, 1 out]
        n162 = call "发送显示帮助信息.vi"("Message Enqueuer"=w231) -> ()  [unwired: 9 in, 2 out]
      }
      event "切换界面": Value Change {
        n163 = event-data() -> ("CtlRef"=w233:refnum<vi>, "NewVal"=w232:bool)  [unwired: 1 in]
        n164 = call "发送切换界面.vi"("界面"=w232, "布尔控件"=w233, "Message Enqueuer"=w234) -> ()  [unwired: 7 in, 2 out]
      }
      event "文本编辑": Key Up {
        # "如果Ctrl键未释放，或者执行释放动作，\n都不执行文本编辑动作，防止Ctrl的组合键失效。"
        n165 = event-data() -> ("ScanCode"=w236:i16)  [unwired: 1 in]
        n166 = call <vilib>:"Intialize Keyboard.vi"() -> ("error out"=w245:errorcluster, "device ID"=w246:refnum<k1>)  [unwired: 10 in]
        n167 = call-poly <vilib>:"Acquire Input Data.vi"("device ID"=w246, "error in (no error)"=w245) -> ("device ID"=w244:refnum<k1>, "keys pressed"=w242:T10, "error out"=w243:errorcluster)  [unwired: 15 in]
        n168 = call-poly <vilib>:"Close Input Device.vi"("error in (no error)"=w243, "device ID"=w244) -> ()  [unwired: 8 in, 1 out]
        n169 = Index Array(array=w242) -> (element=w241:T5)  [unwired: 1 in]
        n170 = Equal?(x=i16 29, y=w236) -> (x = y?=w237:bool)
        n171 = Equal?(x=w241, y=T5."LCONTROL") -> (x = y?=w238:bool)
        n172 = Or(x=w238, y=w237) -> (x .or. y?=w235:bool)
        n173 = case shown="True" w235 {
          tunnel: w248 -> [w251 _]
          tunnel: w247 -> [w250 _]
          tunnel: w236 -> [w249 _]
          frame False {
            n174 = call "发送编辑文本.vi"("error in (no error)"=w250, "扫描代码"=w249, "Message Enqueuer"=w251) -> ()  [unwired: 7 in, 2 out]
          }
          frame True {
          }
        }
      }
    }
  }
  n175 = call <vilib>:"Send Normal Stop.vi"("error in (no error)"=w26, "Message Enqueuer"=w31) -> ()  [unwired: 9 in, 1 out]
  n176 = call <vilib>:"Send Normal Stop.vi"("error in (no error)"=w28, "Message Enqueuer"=w30) -> ()  [unwired: 9 in, 1 out]
